vi "t0 dt (SubVI).vi"(9 "ScaleAbciss":enum16{"Время", "Растояние"}(ring) caption="Ось абсцисс", 10 "speed":dbl=1500.0 caption="скорость звука, м/с", 11 "UNDT_Cluster":T1 {"Gain Coeff" format="%#_6e"; "Reserve 1" format="%02x"; "Mux TX/RX" format="%02x"; "ScanDelay" format="%02x"; "PacketCounter" format="%08x"; "SamplingInterval" format="%#_6e"; "Lose Packet" format="%08x"; "EncodersParam2" format="%016x"; "EncodersParam1" format="%016x"; "CRC 8" format="%02x"; "N chanel" format="%02x"; "N tick" format="%02x"; "Ncycle" format="%04x"; "FrameFormatVersion" format="%02x"; "MagicWord" format="%.0x"}) -> (3 "magnitude":cluster{"t0":dbl, "dt":dbl, "magnitude":dbl[]})   [LabVIEW 2017]
uses:
  Control_EU/UNDT_ClusterPackRevers (Type).ctl
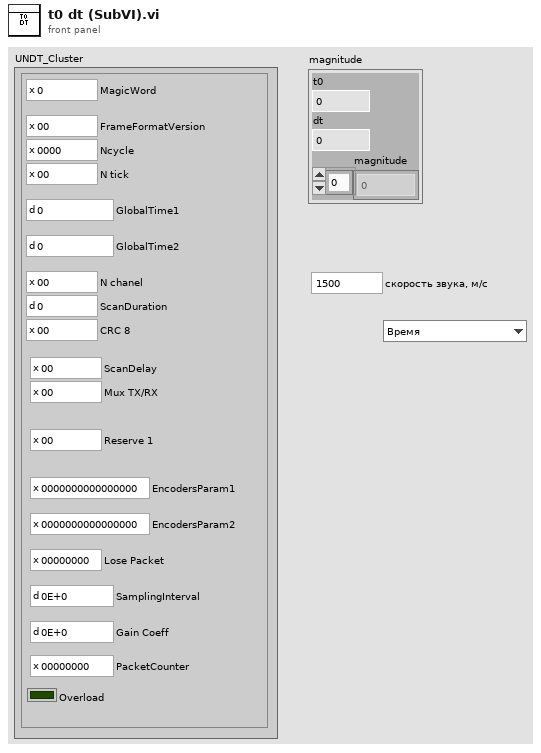
[diagram p1: front panel]
types:
  T1 = typedef "UNDT_ClusterPackRevers (Type).ctl" = cluster{"PacketCounter":u32, "Gain Coeff":sgl, "SamplingInterval":sgl, "Lose Packet":u32, "EncodersParam2":u64, "EncodersParam1":u64, "Reserve 1":u8, "Mux TX/RX":u8, "ScanDelay":u16, "CRC 8":u8, "ScanDuration":u16, "N chanel":u8, "GlobalTime2":u32, "GlobalTime1":u32, "N tick":u8, "Ncycle":u16, "FrameFormatVersion":u8, "MagicWord":u32, "Overload":bool}
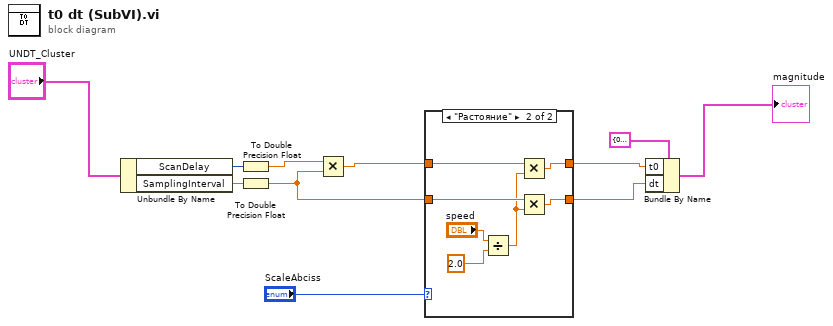
[diagram p0: block diagram]
diagram:
  n1 = Unbundle By Name("UNDT_Cluster") -> ("ScanDelay"=w9:u16, "SamplingInterval"=w10:sgl)
  n2 = To Double Precision Float(number=w9) -> (double precision float=w5:dbl)
  n3 = To Double Precision Float(number=w10) -> (double precision float=w4:dbl)
  n4 = Multiply(x=w5, y=w4) -> (x*y=w2:dbl)
  n5 = case shown="\"Растояние\"" "ScaleAbciss" {
    tunnel: w2 -> [w13 w17]
    tunnel: [w13 w18] -> w1
    tunnel: [w12 w20] -> w3
    tunnel: w4 -> [w12 w19]
    frame "Время", Default {
    }
    frame "Растояние" {
      n6 = Divide(x="speed", y=2.0) -> (x/y=w14:dbl)
      n7 = Multiply(x=w17, y=w14) -> (x*y=w18:dbl)
      n8 = Multiply(x=w19, y=w14) -> (x*y=w20:dbl)
    }
  }
  n9 = Bundle By Name(cluster=cluster{"t0":dbl, "dt":dbl, "magnitude":dbl[]} {"t0"=0.0, "dt"=0.0, "magnitude"=[]} ("magnitude"), "t0"=w1, "dt"=w3) -> (→"magnitude":cluster{"t0":dbl, "dt":dbl, "magnitude":dbl[]})
